vi "Standard Type To Switch State.vi"(1 "Standard Type":T2) -> (0 "Switch State":T1)   [LabVIEW 2023, in "ACM 4509 Cal Standard.lvlib" / "Cal Standard.lvclass"]
uses:
  Cal Standard.lvclass
  Instruments/Cal Standard/Type Definitions/Standard Type.ctl
  Dependencies/ACM/API/Controls/ACM Switch States.ctl
  Dependencies/ACM/ACM Visa Driver.lvlib
  Instruments/RFFixtureCharact.Instruments.lvlib
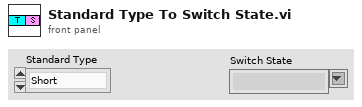
[diagram p1: front panel]
types:
  T1 = typedef "ACM Visa Driver.lvlib/ACM Switch States.ctl" = string
  T2 = typedef "RFFixtureCharact.Instruments.lvlib/Standard Type.ctl" = enum16{"Short", "Open", "Load"}
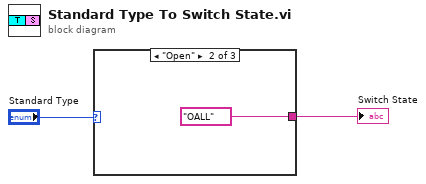
[diagram p0: block diagram]
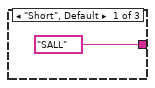
[diagram p2: hidden frame]
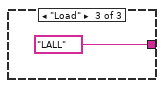
[diagram p3: hidden frame]
diagram:
  n1 = case shown="\"Open\"" "Standard Type" {
    tunnel: [T1 "SALL" ("Standard Type") T1 "OALL" ("Standard Type") T1 "LALL" ("Standard Type")] -> w1
    frame "Short", Default {
    }
    frame "Open" {
    }
    frame "Load" {
    }
  }
  "Switch State" <- w1
